vi "位移信号处理.vi"(8 "位移2":dbl[](graph), 11 "位移1":dbl[](graph)) -> (0 "相位谱 2":dbl[](graph), 1 "幅度谱 2":dbl[](graph), 2 "相位谱":dbl[](graph), 3 "幅度谱":dbl[](graph))   [LabVIEW 2014]
uses:
  <vilib>/Analysis/NI_AALPro.lvlib
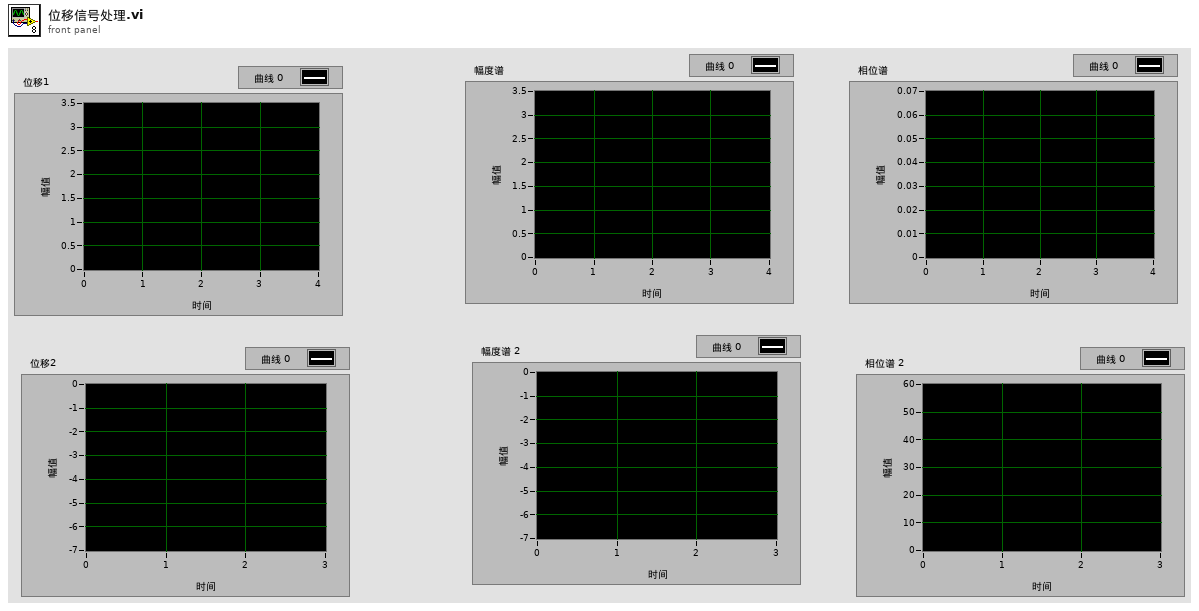
[diagram p1: front panel]
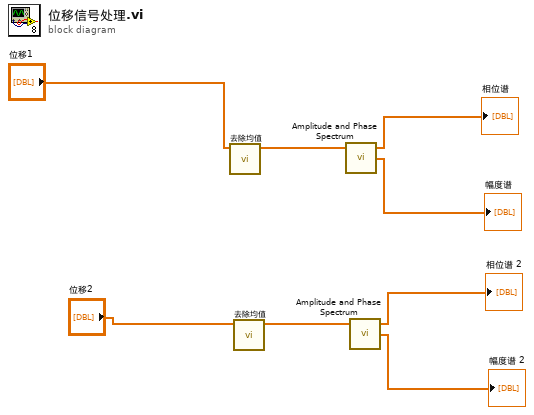
[diagram p0: block diagram]
diagram:
  n1 = call "去除均值.vi"("输入信号"="位移1") -> ("去均值信号"=w6:dbl[])  [unwired: 10 in]
  n2 = call "去除均值.vi"("输入信号"="位移2") -> ("去均值信号"=w5:dbl[])  [unwired: 10 in]
  n3 = call <vilib>:"Amplitude and Phase Spectrum.vi"("Signal (V)"=w6) -> ("Amp Spectrum Phase (radians)"=→"幅度谱":dbl[], "Amp Spectrum Mag (Vrms)"=→"相位谱":dbl[])  [unwired: 2 in, 1 out]
  n4 = call <vilib>:"Amplitude and Phase Spectrum.vi"("Signal (V)"=w5) -> ("Amp Spectrum Phase (radians)"=→"幅度谱 2":dbl[], "Amp Spectrum Mag (Vrms)"=→"相位谱 2":dbl[])  [unwired: 2 in, 1 out]
